vi "setDeviceParameters.vi"(8 "error in (no error)":errorcluster, 11 "OPC in":refnum<class "OPC.lvclass">) -> (0 "error out":errorcluster, 3 "OPC out":refnum<class "OPC.lvclass">)   [LabVIEW 2020, in "OPC.lvclass"]
uses:
  OPC.lvclass
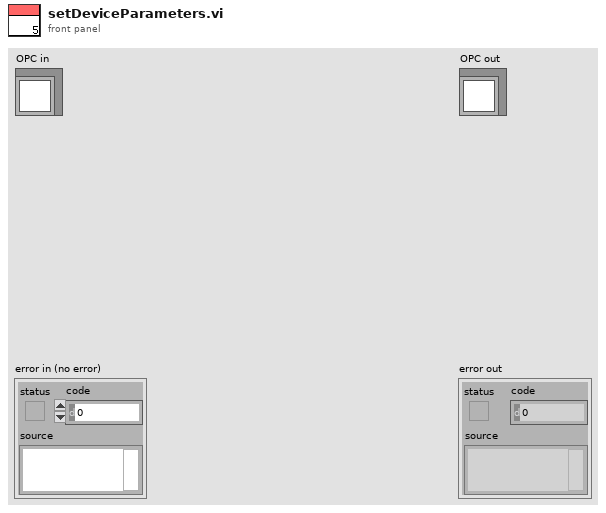
[diagram p1: front panel]
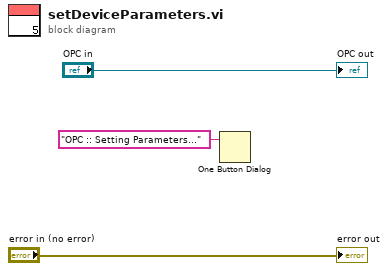
[diagram p0: block diagram]
diagram:
  n1 = One Button Dialog(message="OPC :: Setting Parameters...") -> ()  [unwired: 1 in, 1 out]
  "error out" <- "error in (no error)"
  "OPC out" <- "OPC in"
